vi "Test Newport VI.vi"() -> ()   [LabVIEW 2018]
uses:
  Custom Controls/Group Names.ctl
  Custom Controls/Reference Actions.ctl
  Custom Controls/Reference Sensor.ctl
  Custom Controls/Positioner Names.ctl
  Custom Controls/Queue Data.ctl
  Newport.XPS.CommandInterface
  <vilib>/Utility/cursorutil.llb/Set Cursor (Icon Pict).vi
  Newport.lvlib
panel:
  in  "Stop Button":bool
  in  "Set Speed":dbl caption="Speed (mm/sec)"
  in  "Reverse":bool
  in  "Forward":bool
  in  "Max Position":dbl
  in  "Min Position":dbl
  in  "Set Limits":bool
  out "Current Pos":dbl
  in  "Value":dbl
  in  "Home Offset":bool
  in  "Reboot":bool
  in  "Restart":bool
  in  "All?":bool
  in  "Un-Initialize":bool
  in  "PositionerName":T1
  in  "ReferencingParameter":dbl=2.0 format="%#_13g"
  in  "ReferencingSensor":T2
  in  "ReferencingAction":T3
  in  "Stop Reference":bool
  in  "Start Reference":bool
  in  "Reference":bool
  in  "GroupName":T4
  in  "Initialize":bool
  in  "Absolute Move":bool
  in  "Home":bool
  in  "Close":bool
  out "errstring":string
  out "Version":string
  out "FirmwareVersionGet":i32
  # "JOG"
  # "*After changing the 'Offset Home'\nRestart the application for the new values\nto update the Stages.ini file."
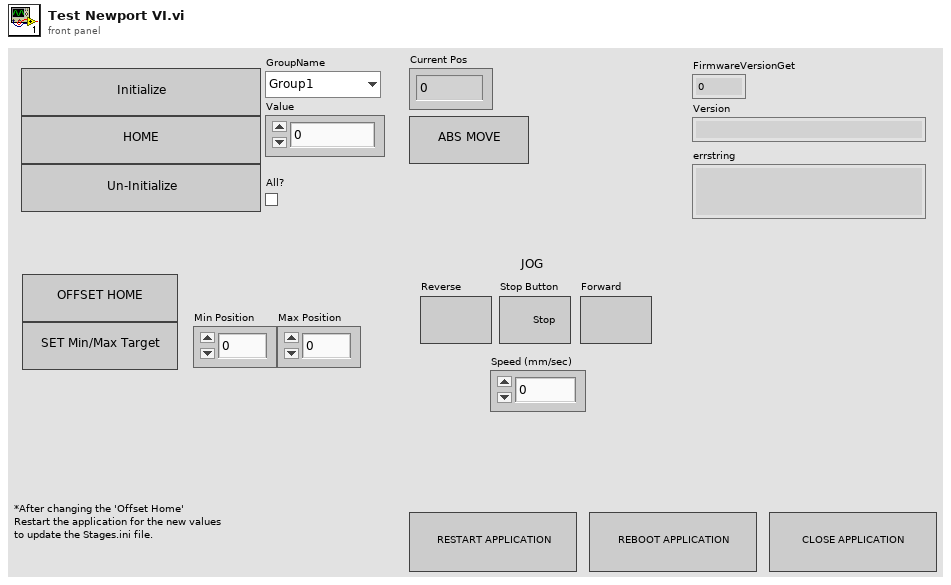
[diagram p1: front panel]
types:
  T1 = typedef "Newport.lvlib/Positioner Names.ctl" = enum16{"Group1.Pos", "Group2.Pos", "Group3.Pos", "Group4.Pos", "Group5.Pos", "Group6.Pos", "Group7.Pos", "Group8.Pos"}
  T2 = typedef "Newport.lvlib/Reference Sensor.ctl" = enum16{"None", "MinusEndOfRun"}
  T3 = typedef "Newport.lvlib/Reference Actions.ctl" = enum16{"LatchOnLowToHighTransition", "SetPosition", "SetPositionToHomePreset", "MoveToPreviouslyLatchedPosition", "MoveRelative"}
  T4 = typedef "Newport.lvlib/Group Names.ctl" = enum16{"Group1", "Group2", "Group3", "Group4", "Group5", "Group6", "Group7", "Group8"}
  T5 = typedef "Newport.lvlib/Queue Data.ctl" = cluster{"State":string, "GroupName":string, "Param Value":dbl}
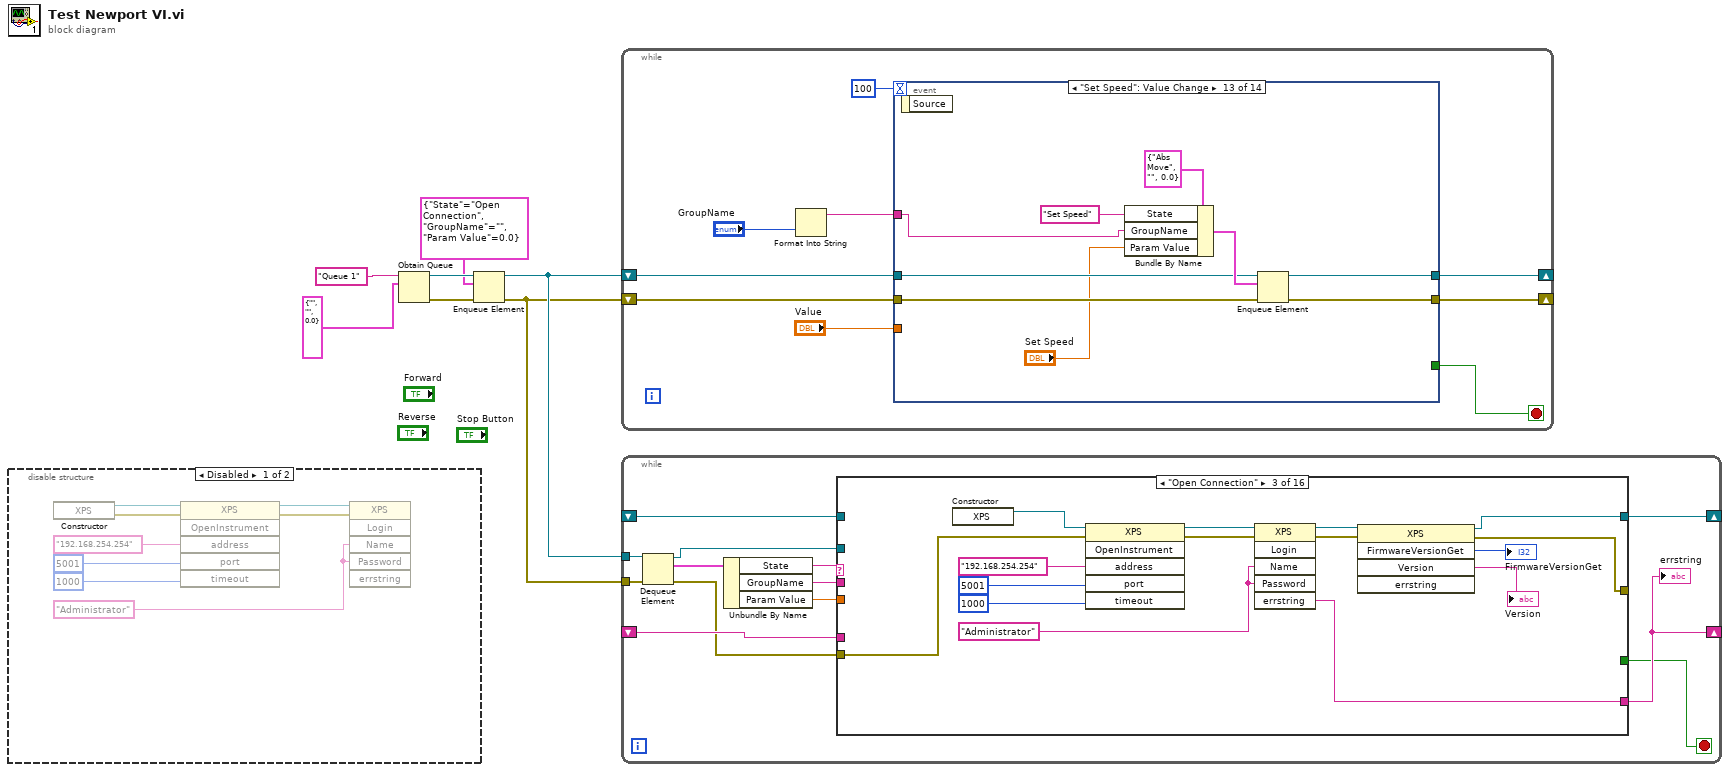
[diagram p0: block diagram]
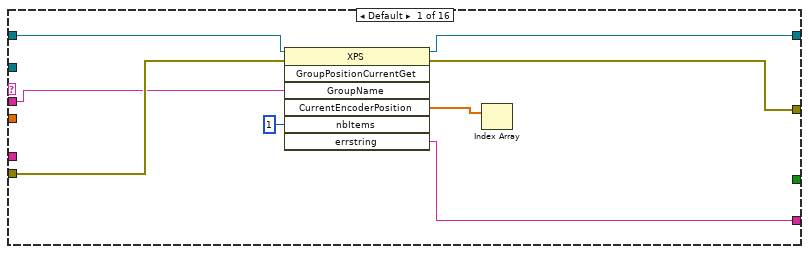
[diagram p3: hidden frame]
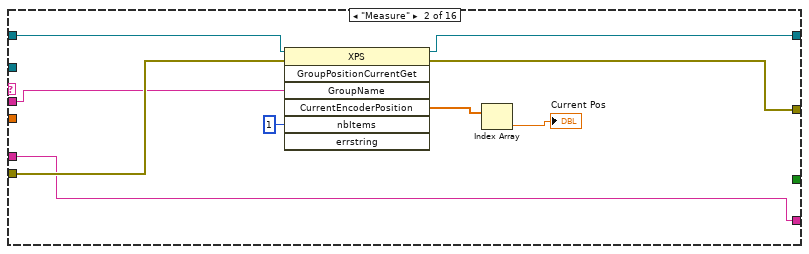
[diagram p4: hidden frame]
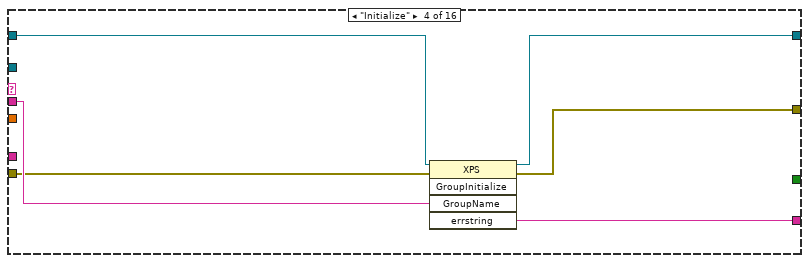
[diagram p5: hidden frame]
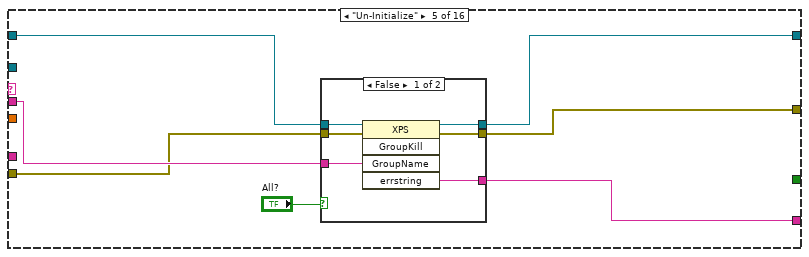
[diagram p6: hidden frame]
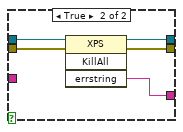
[diagram p7: hidden frame]
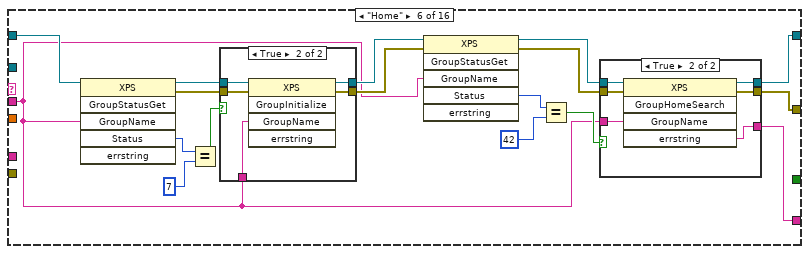
[diagram p8: hidden frame]
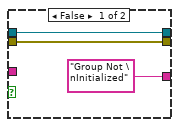
[diagram p10: hidden frame]
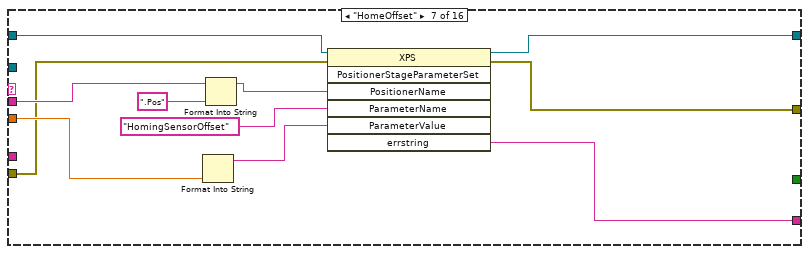
[diagram p11: hidden frame]
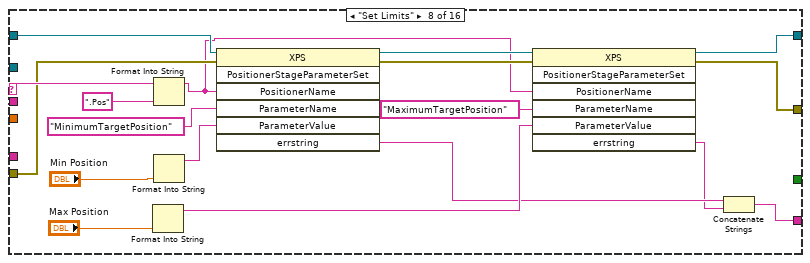
[diagram p12: hidden frame]
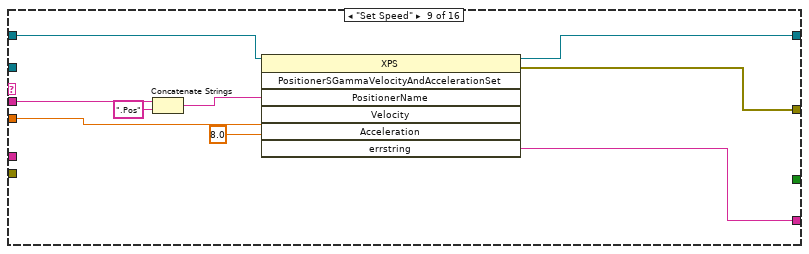
[diagram p13: hidden frame]
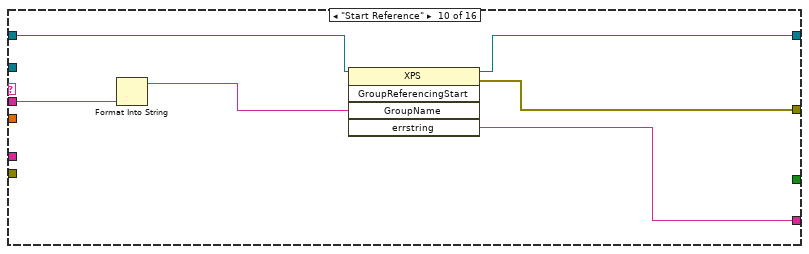
[diagram p14: hidden frame]
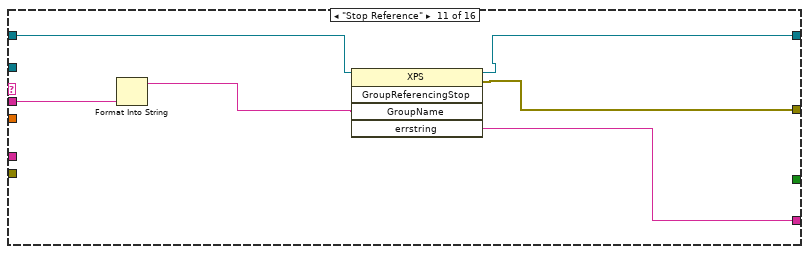
[diagram p15: hidden frame]
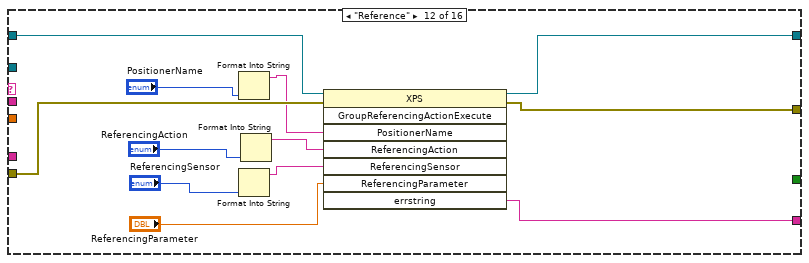
[diagram p16: hidden frame]
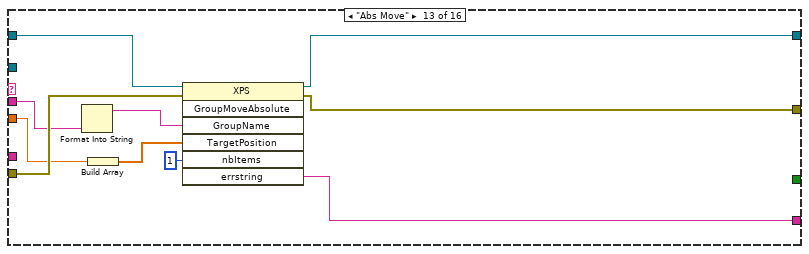
[diagram p17: hidden frame]
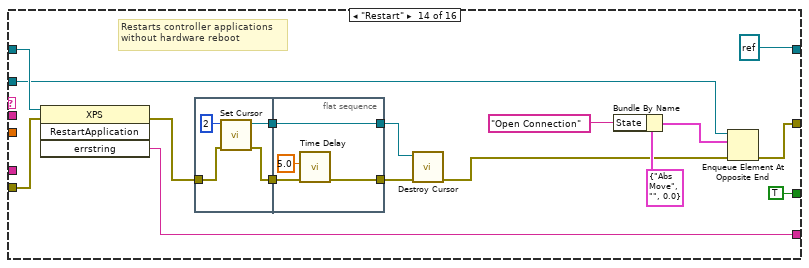
[diagram p18: hidden frame]
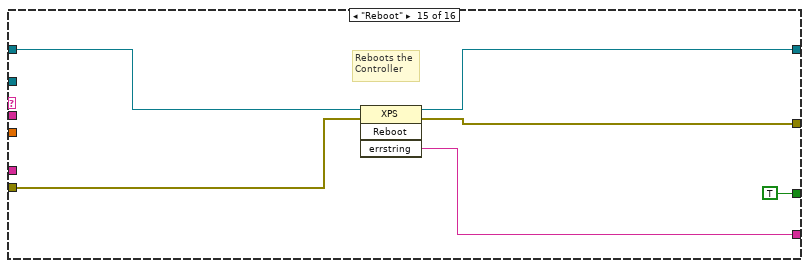
[diagram p19: hidden frame]
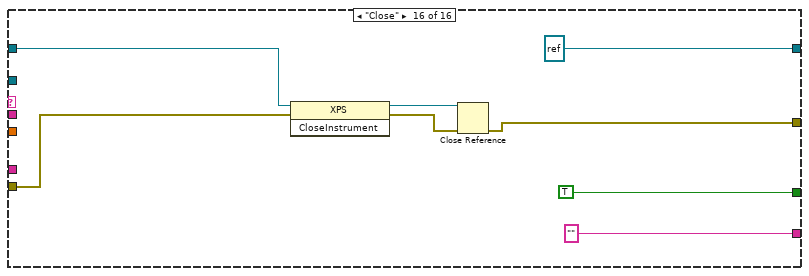
[diagram p20: hidden frame]
diagram:
  n1 = disable-structure shown="Disabled" {
    frame Disabled {
      w11 = "Administrator" ("Name")
      n2 = constructor class="XPS"() -> (reference out=w14:refnum<k24>, error out=w13:errorcluster)  [unwired: 3 in, 1 out]
      n3 = invoke class="XPS" method="OpenInstrument"(reference=w14, error in=w13, "address"="192.168.254.254", "port"=5001, "timeout"=1000) -> (reference out=w15:refnum<k24>, error out=w12:errorcluster)  [unwired: 1 in, 4 out]
      n4 = invoke class="XPS" method="Login"(reference=w15, error in=w12, "Name"=w11, "Password"=w11) -> ()  [unwired: 2 in, 6 out]
    }
    frame Enabled {
    }
  }
  n5 = Obtain Queue(name (unnamed)="Queue 1", element data type=T5 {"State"="", "GroupName"="", "Param Value"=0.0}) -> (queue out=w6:refnum<queue>, error out=w5:errorcluster)  [unwired: 3 in, 1 out]
  n6 = Enqueue Element(queue=w6, element=T5 {"State"="Open Connection", "GroupName"="", "Param Value"=0.0}, error in (no error)=w5) -> (queue out=w4:refnum<queue>, error out=w3:errorcluster)  [unwired: 1 in, 1 out]
  n7 = while {
    shift-right: [w20] -> _
    shift-left: w4 -> [w22]
    shift-right: [w19] -> _
    shift-left: w3 -> [w21]
    stop <- w23 stop-if-true
    n8 = Format Into String("GroupName") -> (resulting string=w18:string)  [unwired: 3 in, 1 out]
    n9 = event shown="[12] \"Set Speed\": Value Change" {
      selector: _ -> [_ _ _ _ _ _ _ _ _ _ _ _ _ _]
      dyn-events: _ -> [_ _ _ _ _ _ _ _ _ _ _ _ _ _]
      timeout: 100 -> [_ _ _ _ _ _ _ _ _ _ _ _ _ _]
      tunnel: [_ _ _ _ _ _ _ _ _ _ _ _ _ TRUE] -> w23
      tunnel: w22 -> [w28 w41 w46 w54 w61 w66 w76 w82 w92 w100 w107 w115 w124 w133]
      tunnel: w21 -> [w26 w40 w45 w53 w59 w65 w75 w81 w91 w103 w106 w114 w123 w136]
      tunnel: [w27 w39 w44 w52 w60 w68 w74 w84 w90 w101 w109 w117 w126 w134] -> w20
      tunnel: [w25 w38 w43 w51 w58 w67 w73 w83 w89 w102 w108 w116 w125 w135] -> w19
      tunnel: w18 -> [w29 w34 w42 w50 _ _ w72 w80 w88 w96 w105 w113 w122 _]
      tunnel: "Value" -> [_ w33 _ _ _ _ _ _ _ _ w104 _ _ _]
      event Timeout {
        n10 = event-data() -> ()  [unwired: 1 in, 1 out]
        n11 = Bundle By Name(cluster=T5 {"State"="Abs Move", "GroupName"="", "Param Value"=0.0}, "State"="Measure", "GroupName"=w29) -> (w32:T5)
        n12 = Enqueue Element(queue=w28, element=w32, error in (no error)=w26) -> (queue out=w27:refnum<queue>, error out=w25:errorcluster)  [unwired: 1 in, 1 out]
      }
      event "Absolute Move": Value Change {
        n13 = event-data() -> ()  [unwired: 1 in, 1 out]
        n14 = Bundle By Name(cluster=T5 {"State"="Abs Move", "GroupName"="", "Param Value"=0.0}, "State"="Abs Move", "GroupName"=w34, "Param Value"=w33) -> (w36:T5)
        n15 = Enqueue Element(queue=w41, element=w36, error in (no error)=w40) -> (queue out=w39:refnum<queue>, error out=w38:errorcluster)  [unwired: 1 in, 1 out]
      }
      event "Initialize": Value Change {
        n16 = event-data() -> ()  [unwired: 1 in, 1 out]
        n17 = Bundle By Name(cluster=T5 {"State"="Abs Move", "GroupName"="", "Param Value"=0.0}, "State"="Initialize", "GroupName"=w42) -> (w49:T5)
        n18 = Enqueue Element(queue=w46, element=w49, error in (no error)=w45) -> (queue out=w44:refnum<queue>, error out=w43:errorcluster)  [unwired: 1 in, 1 out]
      }
      event "Un-Initialize": Value Change {
        n19 = event-data() -> ()  [unwired: 1 in, 1 out]
        n20 = Bundle By Name(cluster=T5 {"State"="Abs Move", "GroupName"="", "Param Value"=0.0}, "State"="Un-Initialize", "GroupName"=w50) -> (w57:T5)
        n21 = Enqueue Element(queue=w54, element=w57, error in (no error)=w53) -> (queue out=w52:refnum<queue>, error out=w51:errorcluster)  [unwired: 1 in, 1 out]
      }
      event "Restart": Value Change {
        n22 = event-data() -> ()  [unwired: 1 in, 1 out]
        n23 = Bundle By Name(cluster=T5 {"State"="Abs Move", "GroupName"="", "Param Value"=0.0}, "State"="Restart") -> (w64:T5)
        n24 = Enqueue Element(queue=w61, element=w64, error in (no error)=w59) -> (queue out=w60:refnum<queue>, error out=w58:errorcluster)  [unwired: 1 in, 1 out]
      }
      event "Reboot": Value Change {
        n25 = event-data() -> ()  [unwired: 1 in, 1 out]
        n26 = Bundle By Name(cluster=T5 {"State"="Abs Move", "GroupName"="", "Param Value"=0.0}, "State"="Reboot") -> (w71:T5)
        n27 = Enqueue Element(queue=w66, element=w71, error in (no error)=w65) -> (queue out=w68:refnum<queue>, error out=w67:errorcluster)  [unwired: 1 in, 1 out]
      }
      event "Start Reference": Value Change {
        n28 = event-data() -> ()  [unwired: 1 in, 1 out]
        n29 = Bundle By Name(cluster=T5 {"State"="Abs Move", "GroupName"="", "Param Value"=0.0}, "State"="Start Reference", "GroupName"=w72) -> (w79:T5)
        n30 = Enqueue Element(queue=w76, element=w79, error in (no error)=w75) -> (queue out=w74:refnum<queue>, error out=w73:errorcluster)  [unwired: 1 in, 1 out]
      }
      event "Reference": Value Change {
        n31 = event-data() -> ()  [unwired: 1 in, 1 out]
        n32 = Bundle By Name(cluster=T5 {"State"="Abs Move", "GroupName"="", "Param Value"=0.0}, "State"="Reference", "GroupName"=w80) -> (w87:T5)
        n33 = Enqueue Element(queue=w82, element=w87, error in (no error)=w81) -> (queue out=w84:refnum<queue>, error out=w83:errorcluster)  [unwired: 1 in, 1 out]
      }
      event "Stop Reference": Value Change {
        n34 = event-data() -> ()  [unwired: 1 in, 1 out]
        n35 = Bundle By Name(cluster=T5 {"State"="Abs Move", "GroupName"="", "Param Value"=0.0}, "State"="Stop Reference", "GroupName"=w88) -> (w95:T5)
        n36 = Enqueue Element(queue=w92, element=w95, error in (no error)=w91) -> (queue out=w90:refnum<queue>, error out=w89:errorcluster)  [unwired: 1 in, 1 out]
      }
      event "Home": Value Change {
        n37 = event-data() -> ()  [unwired: 1 in, 1 out]
        n38 = Bundle By Name(cluster=T5 {"State"="Abs Move", "GroupName"="", "Param Value"=0.0}, "State"="Home" ("element"), "GroupName"=w96) -> (w97:T5)
        n39 = Enqueue Element(queue=w100, element=w97, error in (no error)=w103) -> (queue out=w101:refnum<queue>, error out=w102:errorcluster)  [unwired: 1 in, 1 out]
      }
      event "Home Offset": Value Change {
        n40 = event-data() -> ()  [unwired: 1 in, 1 out]
        n41 = Bundle By Name(cluster=T5 {"State"="Abs Move", "GroupName"="", "Param Value"=0.0}, "State"="HomeOffset" ("element"), "GroupName"=w105, "Param Value"=w104) -> (w112:T5)
        n42 = Enqueue Element(queue=w107, element=w112, error in (no error)=w106) -> (queue out=w109:refnum<queue>, error out=w108:errorcluster)  [unwired: 1 in, 1 out]
      }
      event "Set Limits": Value Change {
        n43 = event-data() -> ()  [unwired: 1 in, 1 out]
        n44 = Bundle By Name(cluster=T5 {"State"="Abs Move", "GroupName"="", "Param Value"=0.0}, "State"="Set Limits" ("element"), "GroupName"=w113) -> (w120:T5)
        n45 = Enqueue Element(queue=w115, element=w120, error in (no error)=w114) -> (queue out=w117:refnum<queue>, error out=w116:errorcluster)  [unwired: 1 in, 1 out]
      }
      event "Set Speed": Value Change {
        n46 = event-data() -> ()  [unwired: 1 in, 1 out]
        n47 = Bundle By Name(cluster=T5 {"State"="Abs Move", "GroupName"="", "Param Value"=0.0}, "State"="Set Speed" ("element"), "GroupName"=w122, "Param Value"="Set Speed") -> (w129:T5)
        n48 = Enqueue Element(queue=w124, element=w129, error in (no error)=w123) -> (queue out=w126:refnum<queue>, error out=w125:errorcluster)  [unwired: 1 in, 1 out]
      }
      event "Close": Value Change {
        n49 = event-data() -> ()  [unwired: 1 in, 1 out]
        n50 = Bundle By Name(cluster=T5 {"State"="Abs Move", "GroupName"="", "Param Value"=0.0}, "State"="Close" ("element")) -> (w130:T5)
        n51 = Enqueue Element(queue=w133, element=w130, error in (no error)=w136) -> (queue out=w134:refnum<queue>, error out=w135:errorcluster)  [unwired: 1 in, 1 out]
      }
    }
  }
  n52 = while {
    tunnel: w4 -> [w150]
    tunnel: w3 -> [w149]
    shift-right: [w147] -> _
    shift-left: _ -> [w148]
    shift-right: [w146] -> _
    shift-left: _ -> [w145]
    stop <- w144 stop-if-true
    n53 = Dequeue Element(queue=w150, error in (no error)=w149) -> (queue out=w138:refnum<queue>, element=w142:T5, error out=w143:errorcluster)  [unwired: 1 in, 1 out]
    n54 = Unbundle By Name(w142) -> ("State"=w141:string, "GroupName"=w140:string, "Param Value"=w139:dbl)
    n55 = case shown="\"Open Connection\"" w141 {
      tunnel: [w151 w159 w171 w188 w195 w220 w244 w251 w272 w279 w285 w299 w309 w325 w337 "" ("errstring")] -> w146
      tunnel: w148 -> [w155 w164 _ w186 w193 w212 w241 w263 w270 w280 w288 w301 w310 w327 w341 w348]
      tunnel: [w156 w165 w172 w187 w194 w223 w240 w258 w269 w281 w287 w298 w306 refnum<k24> refnum ("new reference") w339 refnum<k24> refnum ("new reference")] -> w147
      tunnel: w145 -> [_ w159 _ _ _ _ _ _ _ _ _ _ _ _ _ _]
      tunnel: [_ _ _ _ _ _ _ _ _ _ _ _ _ TRUE TRUE TRUE] -> w144
      tunnel: w143 -> [w154 w163 w176 w183 w190 _ w242 w264 _ _ _ w296 w308 w326 w340 w344]
      tunnel: [w153 w162 w170 w185 w192 w222 w243 w259 w271 w278 w286 w300 w305 w319 w338 w342] -> _
      tunnel: w140 -> [w152 w161 _ w184 w191 w207 w250 w268 w277 w283 w289 _ w307 _ _ _]
      tunnel: w139 -> [_ _ _ _ _ _ w246 _ w274 _ _ _ w303 _ _ _]
      tunnel: w138 -> [_ _ _ _ _ _ _ _ _ _ _ _ _ w320 _ _]
      frame Default {
        n56 = invoke class="XPS" method="GroupPositionCurrentGet"(reference=w155, error in=w154, "GroupName"=w152, "nbItems"=1) -> (reference out=w156:refnum<k24>, error out=w153:errorcluster, "CurrentEncoderPosition"=w157:dbl[], "errstring"=w151:string)  [unwired: 3 in, 3 out]
        n57 = Index Array(array=w157) -> ()  [unwired: 1 in, 1 out]
      }
      frame "Measure" {
        n58 = invoke class="XPS" method="GroupPositionCurrentGet"(reference=w164, error in=w163, "GroupName"=w161, "nbItems"=1) -> (reference out=w165:refnum<k24>, error out=w162:errorcluster, "CurrentEncoderPosition"=w166:dbl[])  [unwired: 3 in, 4 out]
        n59 = Index Array(array=w166) -> (element=→"Current Pos":dbl)  [unwired: 1 in]
      }
      frame "Open Connection" {
        w181 = "Administrator" ("Name")
        n60 = constructor class="XPS"() -> (reference out=w168:refnum<k24>)  [unwired: 3 in, 2 out]
        n61 = invoke class="XPS" method="OpenInstrument"(reference=w168, error in=w176, "address"="192.168.254.254", "port"=5001, "timeout"=1000) -> (reference out=w182:refnum<k24>, error out=w177:errorcluster)  [unwired: 1 in, 4 out]
        n62 = invoke class="XPS" method="Login"(reference=w182, error in=w177, "Name"=w181, "Password"=w181) -> (reference out=w174:refnum<k24>, error out=w169:errorcluster, "errstring"=w171:string)  [unwired: 2 in, 3 out]
        n63 = invoke class="XPS" method="FirmwareVersionGet"(reference=w174, error in=w169) -> (reference out=w172:refnum<k24>, error out=w170:errorcluster, "FirmwareVersionGet"=→"FirmwareVersionGet":i32, "Version"=→"Version":string)  [unwired: 3 in, 1 out]
      }
      frame "Initialize" {
        n64 = invoke class="XPS" method="GroupInitialize"(reference=w186, error in=w183, "GroupName"=w184) -> (reference out=w187:refnum<k24>, error out=w185:errorcluster, "errstring"=w188:string)  [unwired: 2 in, 2 out]
      }
      frame "Un-Initialize" {
        n65 = case shown="False" "All?" {
          tunnel: [w201 w202] -> w195
          tunnel: [w200 w205] -> w194
          tunnel: w193 -> [w199 w206]
          tunnel: [w198 w204] -> w192
          tunnel: w191 -> [w197 _]
          tunnel: w190 -> [w196 w203]
          frame False {
            n66 = invoke class="XPS" method="GroupKill"(reference=w199, error in=w196, "GroupName"=w197) -> (reference out=w200:refnum<k24>, error out=w198:errorcluster, "errstring"=w201:string)  [unwired: 2 in, 2 out]
          }
          frame True {
            n67 = invoke class="XPS" method="KillAll"(reference=w206, error in=w203) -> (reference out=w205:refnum<k24>, error out=w204:errorcluster, "errstring"=w202:string)  [unwired: 2 in, 1 out]
          }
        }
      }
      frame "Home" {
        n68 = invoke class="XPS" method="GroupStatusGet"(reference=w212, "GroupName"=w207) -> (reference out=w213:refnum<k24>, error out=w211:errorcluster, "Status"=w210:i32)  [unwired: 4 in, 3 out]
        n69 = Equal?(x=w210, y=7) -> (x = y?=w208:bool)
        n70 = case shown="True" w208 {
          tunnel: [w225 w230] -> w217
          tunnel: [w224 w229] -> w215
          tunnel: w213 -> [w225 w228]
          tunnel: w211 -> [w224 w227]
          tunnel: w207 -> [_ w226]
          frame False {
          }
          frame True {
            n71 = invoke class="XPS" method="GroupInitialize"(reference=w228, error in=w227, "GroupName"=w226) -> (reference out=w230:refnum<k24>, error out=w229:errorcluster)  [unwired: 2 in, 3 out]
          }
        }
        n72 = invoke class="XPS" method="GroupStatusGet"(reference=w217, error in=w215, "GroupName"=w207) -> (reference out=w216:refnum<k24>, error out=w214:errorcluster, "Status"=w219:i32)  [unwired: 3 in, 3 out]
        n73 = Equal?(x=w219, y=42) -> (x = y?=w221:bool)
        n74 = case shown="True" w221 {
          tunnel: [w233 w239] -> w223
          tunnel: [w232 w238] -> w222
          tunnel: w216 -> [w233 w237]
          tunnel: w214 -> [w232 w236]
          tunnel: w207 -> [_ w235]
          tunnel: ["Group Not \nInitialized" ("y") w234] -> w220
          frame False {
          }
          frame True {
            n75 = invoke class="XPS" method="GroupHomeSearch"(reference=w237, error in=w236, "GroupName"=w235) -> (reference out=w239:refnum<k24>, error out=w238:errorcluster, "errstring"=w234:string)  [unwired: 2 in, 2 out]
          }
        }
      }
      frame "HomeOffset" {
        n76 = Format Into String(w246) -> (resulting string=w245:string)  [unwired: 3 in, 1 out]
        n77 = Format Into String(initial string=w250, ".Pos") -> (resulting string=w248:string)  [unwired: 2 in, 1 out]
        n78 = invoke class="XPS" method="PositionerStageParameterSet"(reference=w241, error in=w242, "PositionerName"=w248, "ParameterName"="HomingSensorOffset", "ParameterValue"=w245) -> (reference out=w240:refnum<k24>, error out=w243:errorcluster, "errstring"=w244:string)  [unwired: 2 in, 4 out]
      }
      frame "Set Limits" {
        n79 = Format Into String("Max Position") -> (resulting string=w254:string)  [unwired: 3 in, 1 out]
        n80 = Format Into String(initial string=w268, ".Pos") -> (resulting string=w257:string)  [unwired: 2 in, 1 out]
        n81 = Format Into String("Min Position") -> (resulting string=w265:string)  [unwired: 3 in, 1 out]
        n82 = invoke class="XPS" method="PositionerStageParameterSet"(reference=w263, error in=w264, "PositionerName"=w257, "ParameterName"="MinimumTargetPosition", "ParameterValue"=w265) -> (reference out=w261:refnum<k24>, error out=w260:errorcluster, "errstring"=w253:string)  [unwired: 2 in, 4 out]
        n83 = invoke class="XPS" method="PositionerStageParameterSet"(reference=w261, error in=w260, "PositionerName"=w257, "ParameterName"="MaximumTargetPosition", "ParameterValue"=w254) -> (reference out=w258:refnum<k24>, error out=w259:errorcluster, "errstring"=w252:string)  [unwired: 2 in, 4 out]
        n84 = Concatenate Strings(w253, w252) -> (w251:string)
      }
      frame "Set Speed" {
        n85 = Concatenate Strings(w277, ".Pos" ("string")) -> (w275:string)
        n86 = invoke class="XPS" method="PositionerSGammaVelocityAndAccelerationSet"(reference=w270, "PositionerName"=w275, "Velocity"=w274, "Acceleration"=8.0) -> (reference out=w269:refnum<k24>, error out=w271:errorcluster, "errstring"=w272:string)  [unwired: 3 in, 4 out]
      }
      frame "Start Reference" {
        n87 = Format Into String(w283) -> (resulting string=w282:string)  [unwired: 3 in, 1 out]
        n88 = invoke class="XPS" method="GroupReferencingStart"(reference=w280, "GroupName"=w282) -> (reference out=w281:refnum<k24>, error out=w278:errorcluster, "errstring"=w279:string)  [unwired: 3 in, 2 out]
      }
      frame "Stop Reference" {
        n89 = Format Into String(w289) -> (resulting string=w284:string)  [unwired: 3 in, 1 out]
        n90 = invoke class="XPS" method="GroupReferencingStop"(reference=w288, "GroupName"=w284) -> (reference out=w287:refnum<k24>, error out=w286:errorcluster, "errstring"=w285:string)  [unwired: 3 in, 2 out]
      }
      frame "Reference" {
        n91 = Format Into String("PositionerName") -> (resulting string=w290:string)  [unwired: 3 in, 1 out]
        n92 = Format Into String("ReferencingSensor") -> (resulting string=w292:string)  [unwired: 3 in, 1 out]
        n93 = Format Into String("ReferencingAction") -> (resulting string=w294:string)  [unwired: 3 in, 1 out]
        n94 = invoke class="XPS" method="GroupReferencingActionExecute"(reference=w301, error in=w296, "PositionerName"=w290, "ReferencingAction"=w294, "ReferencingSensor"=w292, "ReferencingParameter"="ReferencingParameter") -> (reference out=w298:refnum<k24>, error out=w300:errorcluster, "errstring"=w299:string)  [unwired: 2 in, 5 out]
      }
      frame "Abs Move" {
        n95 = Format Into String(w307) -> (resulting string=w304:string)  [unwired: 3 in, 1 out]
        n96 = Build Array(w303) -> (w302:dbl[])
        n97 = invoke class="XPS" method="GroupMoveAbsolute"(reference=w310, error in=w308, "GroupName"=w304, "TargetPosition"=w302, "nbItems"=1) -> (reference out=w306:refnum<k24>, error out=w305:errorcluster, "errstring"=w309:string)  [unwired: 2 in, 4 out]
      }
      frame "Restart" {
        # "Restarts controller applications \nwithout hardware reboot"
        n98 = invoke class="XPS" method="RestartApplication"(reference=w327, error in=w326) -> (error out=w317:errorcluster, "errstring"=w325:string)  [unwired: 2 in, 2 out]
        n99 = flat-sequence {
          tunnel: w317 -> [w330]
          tunnel: [w329] -> w316
          tunnel: [w328] -> w313
          tunnel: [w334] -> w315
          tunnel: w316 -> [w335]
          tunnel: [w333] -> w312
          tunnel: w313 -> [w333]
          frame #0 {
            n100 = call-poly <vilib>:"Set Cursor.vi"("error in (no error)"=w330, "icon"=u16 2) -> ("error out"=w329:errorcluster, "previous cursor ID"=w328:refnum<k1>)  [unwired: 8 in]
          }
          frame #1 {
            n101 = call "Time Delay"("error in (no error)"=w335, "Delay Time (s)"=5.0) -> ("error out"=w334:errorcluster)  [unwired: 9 in]
          }
        }
        n102 = call <vilib>:"Destroy Cursor.vi"("cursor ID"=w312, "error in (no error)"=w315) -> ("error out"=w314:errorcluster)  [unwired: 8 in]
        n103 = Bundle By Name(cluster=T5 {"State"="Abs Move", "GroupName"="", "Param Value"=0.0}, "State"="Open Connection") -> (w321:T5)
        n104 = Enqueue Element At Opposite End(queue=w320, element=w321, error in (no error)=w314) -> (error out=w319:errorcluster)  [unwired: 1 in, 2 out]
      }
      frame "Reboot" {
        # "Reboots the\nController"
        n105 = invoke class="XPS" method="Reboot"(reference=w341, error in=w340) -> (reference out=w339:refnum<k24>, error out=w338:errorcluster, "errstring"=w337:string)  [unwired: 2 in, 1 out]
      }
      frame "Close" {
        n106 = invoke class="XPS" method="CloseInstrument"(reference=w348, error in=w344) -> (reference out=w349:refnum<k24>, error out=w343:errorcluster)  [unwired: 1 in, 1 out]
        n107 = Close Reference(reference=w349, error in (no error)=w343) -> (error out=w342:errorcluster)
      }
    }
    "errstring" <- w146
  }
